vi "DDS.vi"() -> ()   [LabVIEW 2021]
uses:
  <vilib>/RTI DDS Toolkit/Types/RTI DDS Advanced Writer Configuration.ctl
  <vilib>/RTI DDS Toolkit/Types/RTI DDS Advanced Reader Configuration.ctl
  <vilib>/RTI DDS Toolkit/VIs/AdvancedCreateReader_NumI32.vi
  <vilib>/RTI DDS Toolkit/VIs/AdvancedCreateWriter_NumI32.vi
  <vilib>/RTI DDS Toolkit/VIs/Read_NumI32.vi
  <vilib>/RTI DDS Toolkit/VIs/Write_NumI32.vi
  <vilib>/RTI DDS Toolkit/Library/LVDDS_library.lvlib
panel:
  in  "Advanced Reader Configuration 3":T1={"typeName"="std_msgs::msg::dds_::Int32_", "keyName"="", "domainParticipantQoSProfile"="", "dataReaderQoSProfile"="", "forceArrayMapping?"=FALSE, "forceExclusiveReader?"=FALSE, "forceRead? (only ExclusiveReader)"=FALSE, "forceUnboundedString?"=FALSE}
  out "Control Time (ms)":i32
  out "Real Time (ms)":u32
  in  "Advanced Writer Configuration":T2={"typeName"="std_msgs::msg::dds_::Int32_", "keyName"="", "domainParticipantQoSProfile"="", "dataWriterQoSProfile"="", "forceArrayMapping?"=FALSE, "forceUnboundedString?"=FALSE}
  in  "stop":bool
  # "DDS"
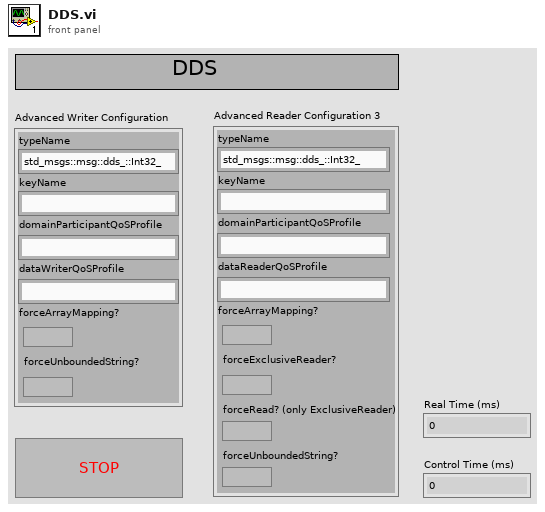
[diagram p1: front panel]
types:
  T1 = typedef "LVDDS_library.lvlib/RTI DDS Advanced Reader Configuration.ctl" = cluster{"typeName":string, "keyName":string, "domainParticipantQoSProfile":string, "dataReaderQoSProfile":string, "forceArrayMapping?":bool, "forceExclusiveReader?":bool, "forceRead? (only ExclusiveReader)":bool, "forceUnboundedString?":bool}
  T2 = typedef "LVDDS_library.lvlib/RTI DDS Advanced Writer Configuration.ctl" = cluster{"typeName":string, "keyName":string, "domainParticipantQoSProfile":string, "dataWriterQoSProfile":string, "forceArrayMapping?":bool, "forceUnboundedString?":bool}
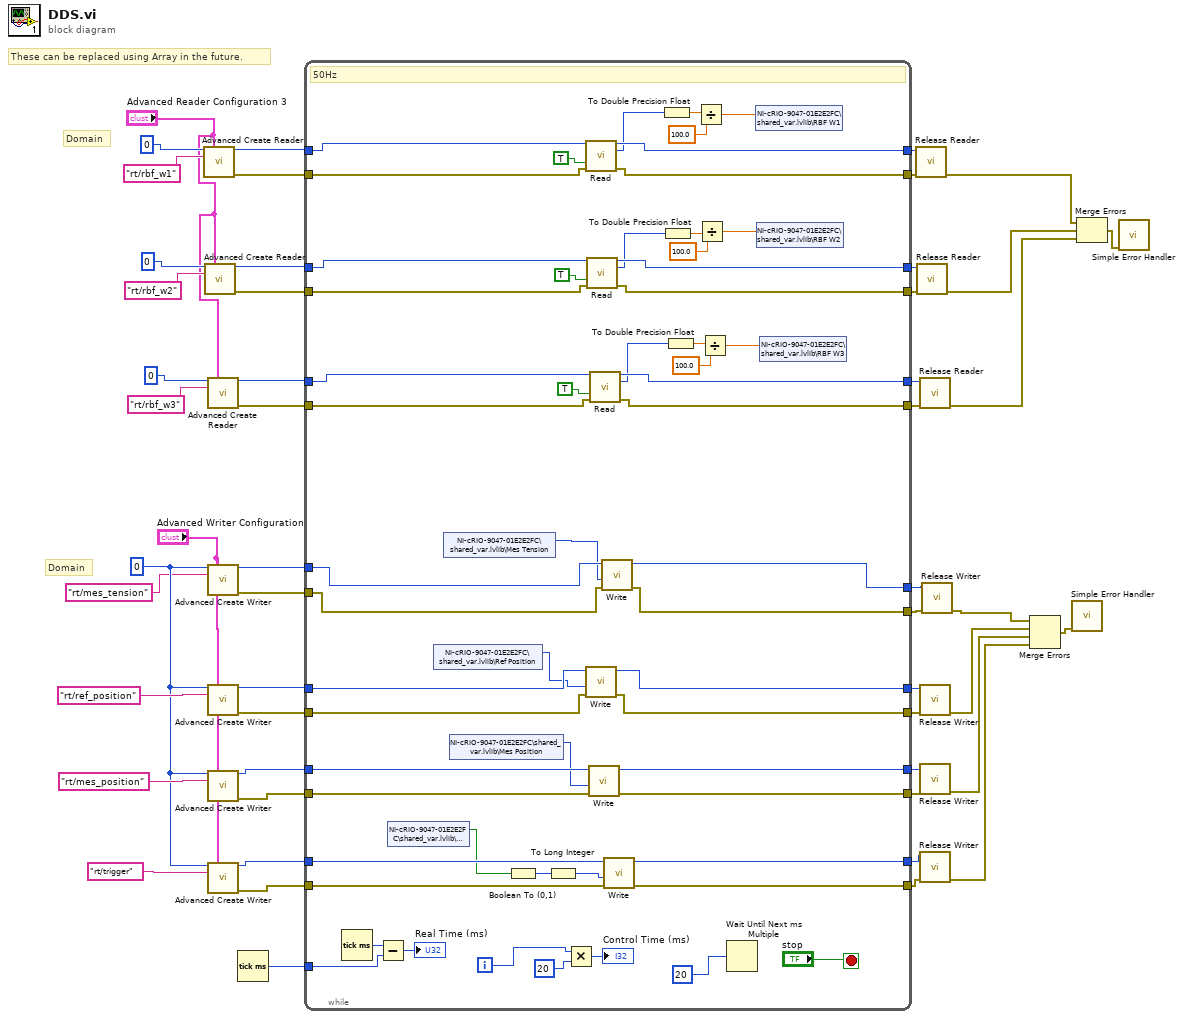
[diagram p0: block diagram]
diagram:
  w20 = u32 0 ("Domain Id")
  # "These can be replaced using Array in the future."
  # "Domain"
  # "Domain"
  n1 = call-poly <vilib>:"Advanced Create Reader.vi"("Domain Id"=u32 0, "Advanced Reader Configuration"="Advanced Reader Configuration 3", "Topic Name"="rt/rbf_w1") -> ("DDS Object Ref"=w8:u64, "error out"=w9:errorcluster)  [unwired: 11 in]
  n2 = call-poly <vilib>:"Advanced Create Reader.vi"("Domain Id"=u32 0, "Advanced Reader Configuration"="Advanced Reader Configuration 3", "Topic Name"="rt/rbf_w2") -> ("DDS Object Ref"=w15:u64, "error out"=w14:errorcluster)  [unwired: 11 in]
  n3 = call-poly <vilib>:"Advanced Create Reader.vi"("Domain Id"=u32 0, "Advanced Reader Configuration"="Advanced Reader Configuration 3", "Topic Name"="rt/rbf_w3") -> ("DDS Object Ref"=w36:u64, "error out"=w37:errorcluster)  [unwired: 11 in]
  n4 = call-poly <vilib>:"Advanced Create Writer.vi"("Domain Id"=w20, "Advanced Writer Configuration"="Advanced Writer Configuration", "Topic Name"="rt/mes_tension") -> ("DDS Object Ref"=w25:u64, "error out"=w24:errorcluster)  [unwired: 11 in]
  n5 = call-poly <vilib>:"Advanced Create Writer.vi"("Domain Id"=w20, "Advanced Writer Configuration"="Advanced Writer Configuration", "Topic Name"="rt/ref_position") -> ("DDS Object Ref"=w31:u64, "error out"=w32:errorcluster)  [unwired: 11 in]
  n6 = call-poly <vilib>:"Advanced Create Writer.vi"("Domain Id"=w20, "Advanced Writer Configuration"="Advanced Writer Configuration", "Topic Name"="rt/mes_position") -> ("DDS Object Ref"=w50:u64, "error out"=w49:errorcluster)  [unwired: 11 in]
  n7 = call-poly <vilib>:"Advanced Create Writer.vi"("Domain Id"=w20, "Advanced Writer Configuration"="Advanced Writer Configuration", "Topic Name"="rt/trigger") -> ("DDS Object Ref"=w42:u64, "error out"=w43:errorcluster)  [unwired: 11 in]
  n8 = Tick Count (ms)() -> (millisecond timer value=w26:u32)
  n9 = while {
    tunnel: w26 -> [w84]
    tunnel: w42 -> [w103]
    tunnel: [w102] -> w41
    tunnel: w43 -> [w104]
    tunnel: [w101] -> w40
    tunnel: w49 -> [w107]
    tunnel: [w105] -> w47
    tunnel: w50 -> [w108]
    tunnel: [w106] -> w48
    tunnel: w32 -> [w96]
    tunnel: [w94] -> w30
    tunnel: w31 -> [w95]
    tunnel: [w93] -> w29
    tunnel: w25 -> [w79]
    tunnel: w24 -> [w78]
    tunnel: [w77] -> w23
    tunnel: [w76] -> w22
    tunnel: w37 -> [w100]
    tunnel: [w97] -> w34
    tunnel: w36 -> [w99]
    tunnel: [w98] -> w35
    tunnel: w14 -> [w65]
    tunnel: [w68] -> w17
    tunnel: w15 -> [w66]
    tunnel: [w67] -> w16
    tunnel: w9 -> [w64]
    tunnel: [w61] -> w6
    tunnel: w8 -> [w63]
    tunnel: [w62] -> w7
    i -> [w83]
    stop <- "stop" stop-if-true
    # "50Hz"
    n10 = Tick Count (ms)() -> (millisecond timer value=w85:u32)
    n11 = Subtract(x=w85, y=w84) -> (x-y=→"Real Time (ms)":u32)
    n12 = shared-variable "NI-cRIO-9047-01E2E2FC\\shared_var.lvlib\\Trigger"() -> (w91:bool)  [unwired: 1 in, 1 out]
    n13 = shared-variable "NI-cRIO-9047-01E2E2FC\\shared_var.lvlib\\Ref Position"() -> (w74:i32)  [unwired: 1 in, 1 out]
    n14 = shared-variable "NI-cRIO-9047-01E2E2FC\\shared_var.lvlib\\Mes Tension"() -> (w75:i32)  [unwired: 1 in, 1 out]
    n15 = shared-variable "NI-cRIO-9047-01E2E2FC\\shared_var.lvlib\\Mes Position"() -> (w88:i32)  [unwired: 1 in, 1 out]
    n16 = Boolean To (0,1)(Boolean=w91) -> (0, 1=w90:i16)
    n17 = To Long Integer(number=w90) -> (32bit integer=w89:i32)
    n18 = Multiply(x=w83, y=20) -> (x*y=→"Control Time (ms)":i32)
    n19 = call-poly <vilib>:"Read.vi"("DDS Object Ref in"=w63, "Only New Samples"=TRUE, "error in (no error)"=w64) -> ("DDS Object Ref out"=w62:u64, "Data"=w56:i32, "error out"=w61:errorcluster)  [unwired: 8 in, 2 out]
    n20 = call-poly <vilib>:"Write.vi"("error in (no error)"=w96, "Data"=w74, "DDS Object Ref in"=w95) -> ("error out"=w94:errorcluster, "DDS Object Ref out"=w93:u64)  [unwired: 7 in]
    n21 = call-poly <vilib>:"Read.vi"("DDS Object Ref in"=w66, "Only New Samples"=TRUE, "error in (no error)"=w65) -> ("DDS Object Ref out"=w67:u64, "Data"=w57:i32, "error out"=w68:errorcluster)  [unwired: 8 in, 2 out]
    n22 = call-poly <vilib>:"Write.vi"("error in (no error)"=w107, "Data"=w88, "DDS Object Ref in"=w108) -> ("error out"=w105:errorcluster, "DDS Object Ref out"=w106:u64)  [unwired: 7 in]
    n23 = call-poly <vilib>:"Read.vi"("DDS Object Ref in"=w99, "Only New Samples"=TRUE, "error in (no error)"=w100) -> ("DDS Object Ref out"=w98:u64, "Data"=w55:i32, "error out"=w97:errorcluster)  [unwired: 8 in, 2 out]
    n24 = call-poly <vilib>:"Write.vi"("error in (no error)"=w78, "Data"=w75, "DDS Object Ref in"=w79) -> ("error out"=w76:errorcluster, "DDS Object Ref out"=w77:u64)  [unwired: 7 in]
    n25 = call-poly <vilib>:"Write.vi"("error in (no error)"=w104, "Data"=w89, "DDS Object Ref in"=w103) -> ("error out"=w101:errorcluster, "DDS Object Ref out"=w102:u64)  [unwired: 7 in]
    n26 = To Double Precision Float(number=w56) -> (double precision float=w59:dbl)
    n27 = To Double Precision Float(number=w57) -> (double precision float=w70:dbl)
    n28 = To Double Precision Float(number=w55) -> (double precision float=w73:dbl)
    n29 = Divide(x=w59, y=100.0) -> (x/y=w54:dbl)
    n30 = Divide(x=w70, y=100.0) -> (x/y=w53:dbl)
    n31 = Divide(x=w73, y=100.0) -> (x/y=w52:dbl)
    n32 = Wait Until Next ms Multiple(millisecond multiple=u32 20) -> ()  [unwired: 1 out]
    n33 = shared-variable "NI-cRIO-9047-01E2E2FC\\shared_var.lvlib\\RBF W1"(w54) -> ()  [unwired: 1 in, 1 out]
    n34 = shared-variable "NI-cRIO-9047-01E2E2FC\\shared_var.lvlib\\RBF W2"(w53) -> ()  [unwired: 1 in, 1 out]
    n35 = shared-variable "NI-cRIO-9047-01E2E2FC\\shared_var.lvlib\\RBF W3"(w52) -> ()  [unwired: 1 in, 1 out]
  }
  n36 = call <vilib>:"Release Reader.vi"("error in (no error)"=w6, "DDS Object Ref"=w7) -> ("error out"=w2:errorcluster)  [unwired: 9 in]
  n37 = call <vilib>:"Release Reader.vi"("error in (no error)"=w17, "DDS Object Ref"=w16) -> ("error out"=w3:errorcluster)  [unwired: 9 in]
  n38 = call <vilib>:"Release Reader.vi"("error in (no error)"=w34, "DDS Object Ref"=w35) -> ("error out"=w4:errorcluster)  [unwired: 9 in]
  n39 = call <vilib>:"Release Writer.vi"("error in (no error)"=w30, "DDS Object Ref"=w29) -> ("error out"=w28:errorcluster)  [unwired: 9 in]
  n40 = call <vilib>:"Release Writer.vi"("error in (no error)"=w47, "DDS Object Ref"=w48) -> ("error out"=w46:errorcluster)  [unwired: 9 in]
  n41 = call <vilib>:"Release Writer.vi"("error in (no error)"=w40, "DDS Object Ref"=w41) -> ("error out"=w33:errorcluster)  [unwired: 9 in]
  n42 = call <vilib>:"Release Writer.vi"("error in (no error)"=w22, "DDS Object Ref"=w23) -> ("error out"=w18:errorcluster)  [unwired: 9 in]
  n43 = Merge Errors(w18, w28, w46, w33) -> (w45:errorcluster)
  n44 = call <vilib>:"Simple Error Handler.vi"("error in (no error)"=w45) -> ()  [unwired: 4 in, 5 out]
  n45 = Merge Errors(w2, w3, w4) -> (w5:errorcluster)
  n46 = call <vilib>:"Simple Error Handler.vi"("error in (no error)"=w5) -> ()  [unwired: 4 in, 5 out]
